vi "Create New Element.vi"(8 "error in":errorcluster, 10 "Owner Document":refnum<k20>, 11 "Element in":refnum<class "Element.lvclass">) -> (0 "error out":errorcluster, 3 "Element out":refnum<class "Element.lvclass">)   [LabVIEW 2014, in "Element.lvclass"]
doc: "This vi is used to create an element with all the characteristics and properties that the element has. This vi should be used when saving a new xml document and the elements need to be created. The elements should be linked (parent child relationships given) after using this vi and before the xml document is saved."
uses:
  Element.lvclass
  <resource>/objmgr/DOMUserDefRef.rc
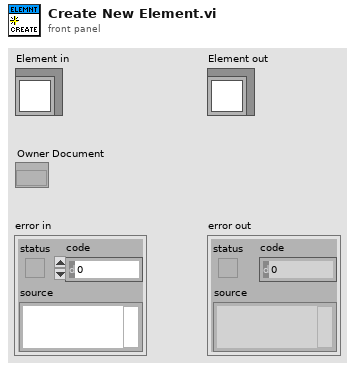
[diagram p1: front panel]
types:
  T1 = typedef "Attribute.ctl" = cluster{"Name":string, "Value":string}
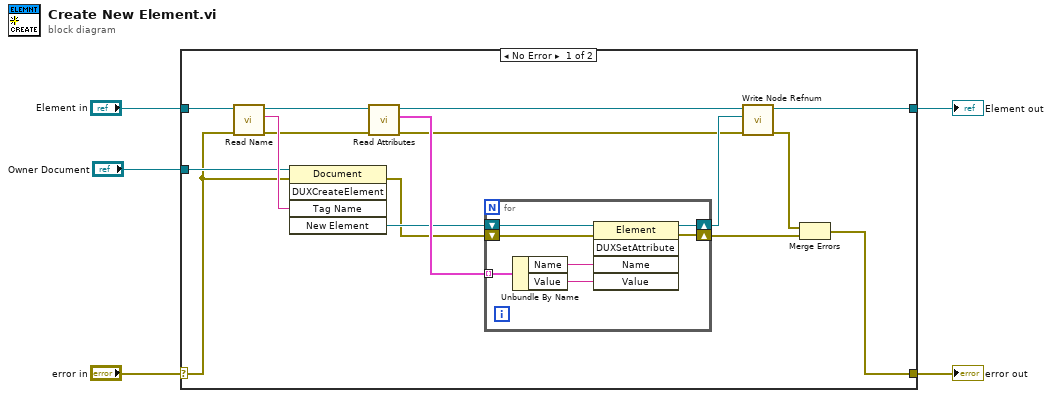
[diagram p0: block diagram]
diagram:
  n1 = case shown="No Error" "error in" {
    selector: "error in" -> [w12 w30]
    tunnel: [w11 w30] -> w4
    tunnel: [w9 w29] -> w2
    tunnel: "Element in" -> [w21 w29]
    tunnel: "Owner Document" -> [w14 _]
    frame No Error {
      n2 = call-dynamic "Read Name.vi"("error in"=w12, "Element in"=w21) -> ("error out"=w15:errorcluster, "Name"=w19:string, "Element out"=w20:refnum<class "Element.lvclass">)  [unwired: 7 in]
      n3 = invoke class="Document" method="DUXCreateElement"(reference=w14, error in=w12, "Tag Name"=w19) -> (error out=w16:errorcluster, "New Element"=w17:refnum<k20>)  [unwired: 2 in, 3 out]
      n4 = call-dynamic "Read Attributes.vi"("error in (no error)"=w15, "Element in"=w20) -> ("error out"=w7:errorcluster, "Attributes"=w18:T1[], "Element out"=w10:refnum<class "Element.lvclass">)  [unwired: 7 in]
      n5 = for {
        tunnel: w18 -> [w26] mode=indexing
        shift-right: [w27] -> w8
        shift-left: w17 -> [w28]
        shift-right: [w22] -> w13
        shift-left: w16 -> [w23]
        n6 = Unbundle By Name(w26) -> ("Name"=w25:string, "Value"=w24:string)
        n7 = invoke class="Element" method="DUXSetAttribute"(reference=w28, error in=w23, "Name"=w25, "Value"=w24) -> (reference out=w27:refnum<k20>, error out=w22:errorcluster)  [unwired: 1 in, 3 out]
      }
      n8 = call-dynamic "Write Node Refnum.vi"("error in"=w7, "Node Refnum"=w8, "Node in"=w10) -> ("error out"=w6:errorcluster, "Node out"=w9:refnum<class "Element.lvclass">)  [unwired: 7 in]
      n9 = Merge Errors(w6, w13) -> (w11:errorcluster)
    }
    frame Error {
    }
  }
  "error out" <- w4
  "Element out" <- w2
